vi "CSM - LogMem.vi"(5 "Init State(\"Macro: Initialize\")":string="Macro: Initialize", 7 "Name(\"\" to use uuid)":string="CSM Tiny") -> ()   [LabVIEW 2020]
doc: "Template for building CSM Module without User Interface.\n\n<b>Inputs:</b>\n- <b>Name(\"\" to use uuid)</b>: Module Name\n - If Input is \"\", an uuid will be used for module name. The module is marked as stand-alone mode and will not be included in module list.\n - Fi Input end with '#', the module will worked in worker mode. Modules with the same name will shared the same message queue. Any external message will be processed by one of the modules, depends on who is free.\n - Otherwise, the input string will be used as module name, which should be unique in system. CSM will go to \"Critical Error\" state if duplicated module name is used in system.\n\n<b>Outputs:</b>\n - N/A"
uses:
  <userlib>/_NEVSTOP/Communicable State Machine(CSM)/_Support/Priority Queue/Priority Queue.lvclass/Priority Queue.ctl
  Typedef/Def - Parsed CSMLog Line - Cluster.ctl
  ad4abf47-66ac-4882-9a91-90711142f294.vi
  aef905fb-f936-4b34-a29e-bd534a28b448.vi
  2c41bf92-7bf3-4770-9d59-94bc44f1e033.vi
  488b24ec-a7c0-4bee-a5e9-5f8eec7386e2.vi
  <userlib>/_NEVSTOP/Communicable State Machine(CSM)/_Support/Process/CSMP-Async Call.vi
  <userlib>/_NEVSTOP/Communicable State Machine(CSM)/_Support/GlobalEvent/GEvt-Generate Status Log.vi
  <userlib>/_NEVSTOP/Communicable State Machine(CSM)/_Support/Process/CSMP-Broadcast.vi
  <userlib>/_NEVSTOP/Communicable State Machine(CSM)/_Support/GlobalEvent/GEvt-Generate Interrupt Log.vi
  <userlib>/_NEVSTOP/Communicable State Machine(CSM)/_Support/GlobalEvent/GEvt-Generate Register Log.vi
  <userlib>/_NEVSTOP/Communicable State Machine(CSM)/_Support/Process/CSMP-Register Status.vi
  <userlib>/_NEVSTOP/Communicable State Machine(CSM)/_Support/GlobalEvent/GEvt-Generate Unregister Log.vi
  <userlib>/_NEVSTOP/Communicable State Machine(CSM)/_Support/Process/CSMP-Unregister Status.vi
  <userlib>/_NEVSTOP/Communicable State Machine(CSM)/_Support/Process/CSMP-Sync Call.vi
  <userlib>/_NEVSTOP/Communicable State Machine(CSM)/_Support/CSMQ/_CSMObj-Unlock.vi
  <userlib>/_NEVSTOP/Communicable State Machine(CSM)/_Support/Process/CSMP-PostPostMsg.vi
  <userlib>/_NEVSTOP/Communicable State Machine(CSM)/_Support/Process/CSMP-PostSendMsg.vi
  <userlib>/_NEVSTOP/Communicable State Machine(CSM)/_Support/CSMQ/_CSMObj-Lock State.vi
  <userlib>/_NEVSTOP/Communicable State Machine(CSM)/_Support/Common/Splite Reason String Part.vi
  <userlib>/_NEVSTOP/Communicable State Machine(CSM)/_Support/Common/Trim Single line Text.vi
  <userlib>/_NEVSTOP/Communicable State Machine(CSM)/_Support/CSMQ/_CSMOFGV Release.vi
  <userlib>/_NEVSTOP/Communicable State Machine(CSM)/_Support/Common/Remove Comments from Line.vi
  <userlib>/_NEVSTOP/Communicable State Machine(CSM)/_Support/Common/Splite Single-line Message.vi
  <userlib>/_NEVSTOP/Communicable State Machine(CSM)/_Support/Common/Parse Next Single-line State.vi
  <userlib>/_NEVSTOP/Communicable State Machine(CSM)/_Support/CSMQ/_CSMOFGV Dequeue.vi
  <userlib>/_NEVSTOP/Communicable State Machine(CSM)/_Support/CSMQ/_CSMObj-Log Error if in a Remote Session.vi
  <userlib>/_NEVSTOP/Communicable State Machine(CSM)/_Support/GlobalEvent/GEvt-Generate State Change Log.vi
  <userlib>/_NEVSTOP/Communicable State Machine(CSM)/_Support/GlobalEvent/GEvt-Generate Remaining States Log.vi
  <userlib>/_NEVSTOP/Communicable State Machine(CSM)/_Support/GlobalEvent/GEvt-Generate Module Destroyed Log.vi
  <userlib>/_NEVSTOP/Communicable State Machine(CSM)/_Support/GlobalEvent/GEvt-Generate Complete Log.vi
  <userlib>/_NEVSTOP/Communicable State Machine(CSM)/_Support/GlobalEvent/GEvt-Generate Module Created Log.vi
  <userlib>/_NEVSTOP/Communicable State Machine(CSM)/_Support/Common/Format Timestamp.vi
  <userlib>/_NEVSTOP/Communicable State Machine(CSM)/AdvanceAPI/CSM - Revert Arguments-Safe String.vi
  <userlib>/_NEVSTOP/Communicable State Machine(CSM)/AdvanceAPI/CSM - Make String Arguments Safe.vi
  <userlib>/_NEVSTOP/Communicable State Machine(CSM)/AdvanceAPI/CSM - Break Down Multiple States String.vi
  <userlib>/_NEVSTOP/Communicable State Machine(CSM)/AdvanceAPI/CSM - Compact Multiple States.vi
  <userlib>/_NEVSTOP/Communicable State Machine(CSM)/_Support/CSMQ/_CSMObj-Message Check.vi
  <userlib>/_NEVSTOP/Communicable State Machine(CSM)/_Support/CSMQ/_CSMObj-Enqueue Cross-Module Message.vi
  <userlib>/_NEVSTOP/Communicable State Machine(CSM)/_Support/CSMQ/_CSMOFGV Get.vi
  <userlib>/_NEVSTOP/Communicable State Machine(CSM)/_Support/FGV-BroadcastRegistry/Cache-Broadcast Registry Search Result.vi
  <userlib>/_NEVSTOP/Communicable State Machine(CSM)/AdvanceAPI/CSM - Register Status Change.vi
  <userlib>/_NEVSTOP/Communicable State Machine(CSM)/AdvanceAPI/CSM - Unregister Status Change.vi
  <userlib>/_NEVSTOP/Communicable State Machine(CSM)/_Support/Common/Hex Str to U8 Data.vi
  <userlib>/_NEVSTOP/Communicable State Machine(CSM)/_Support/Common/Concatenate State with Arguments.vi
  <userlib>/_NEVSTOP/Communicable State Machine(CSM)/_Support/Common/U8 Data to Hex Str.vi
  <userlib>/_NEVSTOP/Communicable State Machine(CSM)/_Support/Priority Queue/Dequeue Element.vi
  <userlib>/_NEVSTOP/Communicable State Machine(CSM)/AdvanceAPI/CSM - Keywords.vi
  <userlib>/_NEVSTOP/Communicable State Machine(CSM)/_Support/Priority Queue/Enqueue Element.vi
  <userlib>/_NEVSTOP/Communicable State Machine(CSM)/Utility/Trim Both Whitespace.vi
  <userlib>/_NEVSTOP/Communicable State Machine(CSM)/_Support/GlobalEvent/FGV-GlobalEventRef.vi
  <userlib>/_NEVSTOP/Communicable State Machine(CSM)/_Support/CSMQ/_CSMOFGV Obtain.vi
  <userlib>/_NEVSTOP/Communicable State Machine(CSM)/_Support/CSMQ/_CSMOFGV.vi
  <userlib>/_NEVSTOP/Communicable State Machine(CSM)/_Support/Error/CSM Not Allowed Message.vi
  <userlib>/_NEVSTOP/Communicable State Machine(CSM)/_Support/GlobalEvent/FGV-StatusChangeEventRef.vi
  <userlib>/_NEVSTOP/Communicable State Machine(CSM)/_Support/FGV-BroadcastRegistry/global-CSMQ FGV Change Flag.vi
  <userlib>/_NEVSTOP/Communicable State Machine(CSM)/_Support/FGV-BroadcastRegistry/global-Broadcast Cache Change Flag.vi
  <userlib>/_NEVSTOP/Communicable State Machine(CSM)/_Support/BroadcastRegistry/HelperVI/Broadcast Item Key.vi
  <userlib>/_NEVSTOP/Communicable State Machine(CSM)/_Support/FGV-BroadcastRegistry/FGV-BroadcastRegistry.vi
  <userlib>/_NEVSTOP/Communicable State Machine(CSM)/_Support/Message/Parse Register Message.vi
  <userlib>/_NEVSTOP/Communicable State Machine(CSM)/_Support/Message/Parse Unregister Message.vi
  <userlib>/_NEVSTOP/Communicable State Machine(CSM)/addons/API-String-Arugments-Support/_Support/Convert API String Arguments to Data(variant).vi
  <userlib>/_NEVSTOP/Communicable State Machine(CSM)/addons/MassData-Parameter/_support/FGV-MassData.vi
  <userlib>/_NEVSTOP/Communicable State Machine(CSM)/addons/API-String-Arugments-Support/_Support/Data To API String Arguments.vi
  <userlib>/_NEVSTOP/Communicable State Machine(CSM)/Communicable State Machine.lvlib
  <userlib>/_NEVSTOP/Communicable State Machine(CSM)/addons/Loop-Support/CSM Loop Support.lvlib
panel:
  out "size(s)":i32
  out "temp":string[](array[string])
  out "Snippets Count":i32
  out "State History":string
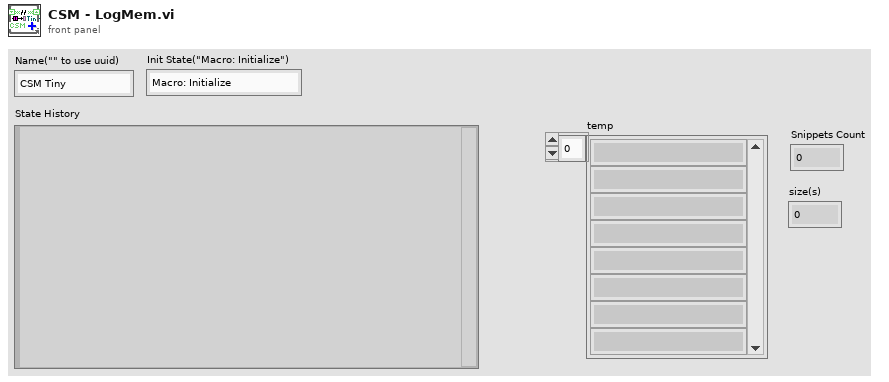
[diagram p1: front panel]
types:
  T1 = enum32{"Invalid", "Standard", "Closed", "Hidden", "Minimized", "Maximized"}
  T2 = enum32{"invalid app kind", "Development System", "Run Time System", "Student Edition", "Embedded LabVIEW", "Evaluation", "Custom"}
  T3 = typedef "Def - Parsed CSMLog Line - Cluster.ctl" = cluster{"Timestamp":timestamp, "Log Type":string, "CSM":string, "Log":string, "RawString":string}
  T4 = typedef "Communicable State Machine.lvlib/_CSM_Response Source Message.ctl" = cluster{"‘State":string, "’Arguments":string, "’Error":errorcluster}
  T5 = cluster{"Core":cluster{"Current VI Reference":refnum<vi>, "Close Panel on Exit?":bool}, "temp":string[], "Snippets Count":i32, "data":T3[]}
  T6 = cluster{"Current VI Reference":refnum<vi>, "Close Panel on Exit?":bool}
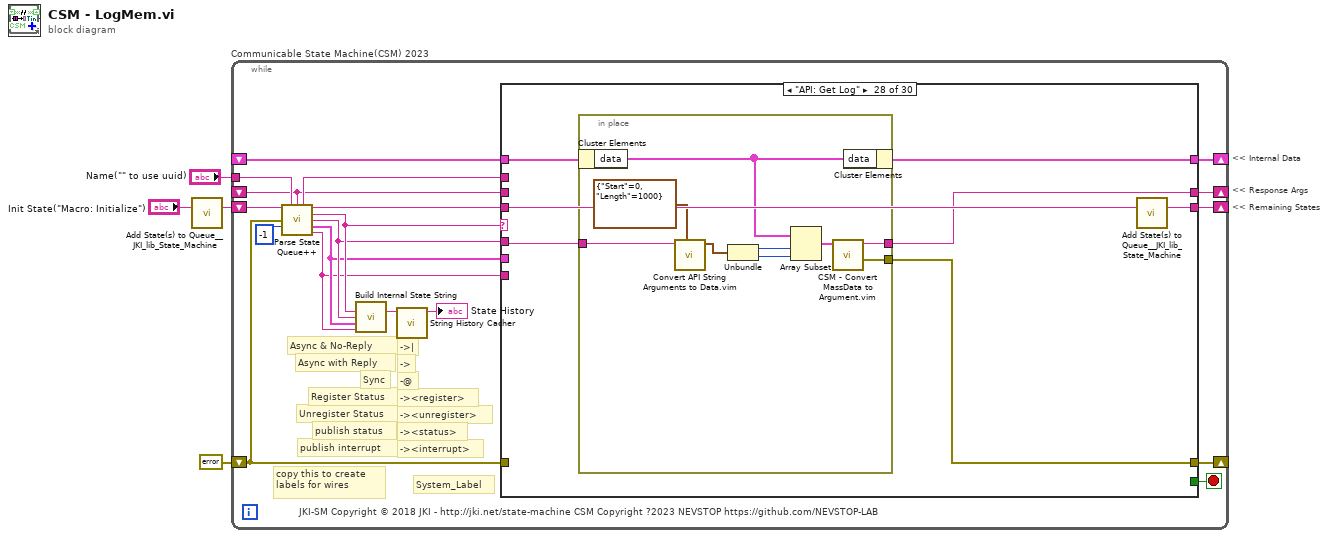
[diagram p0: block diagram]
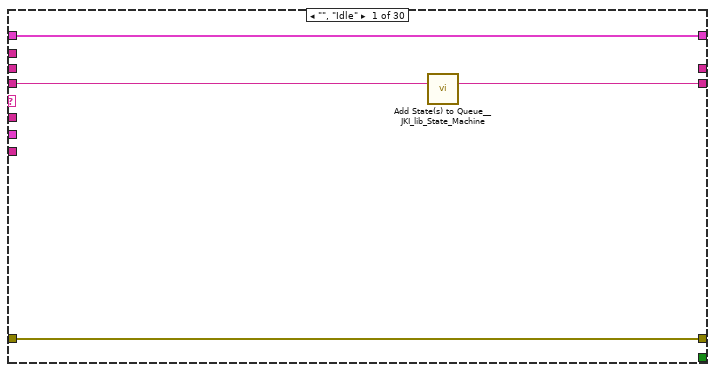
[diagram p2: hidden frame]
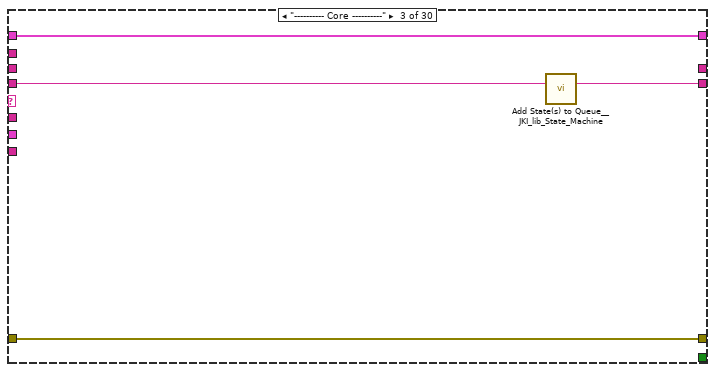
[diagram p4: hidden frame]
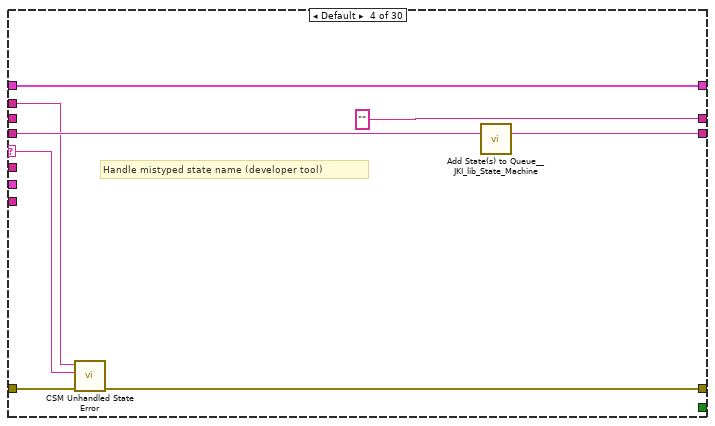
[diagram p5: hidden frame]
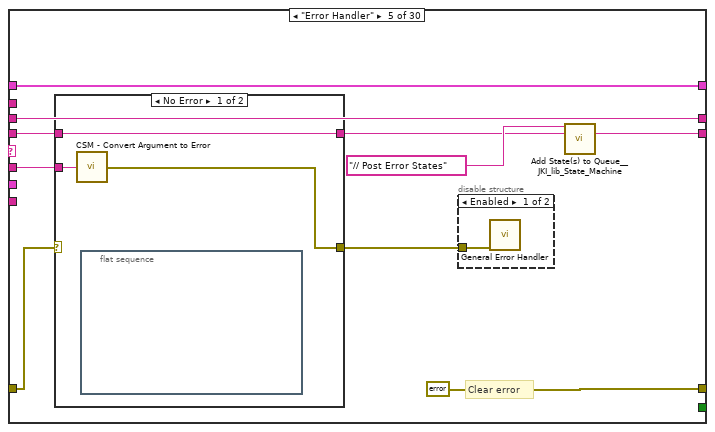
[diagram p6: hidden frame]
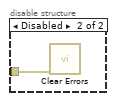
[diagram p7: hidden frame]
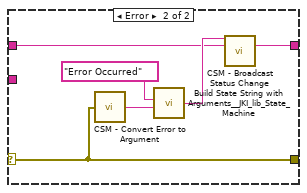
[diagram p8: hidden frame]
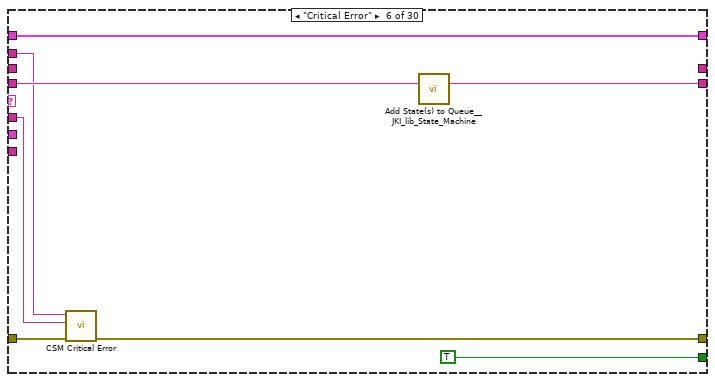
[diagram p9: hidden frame]
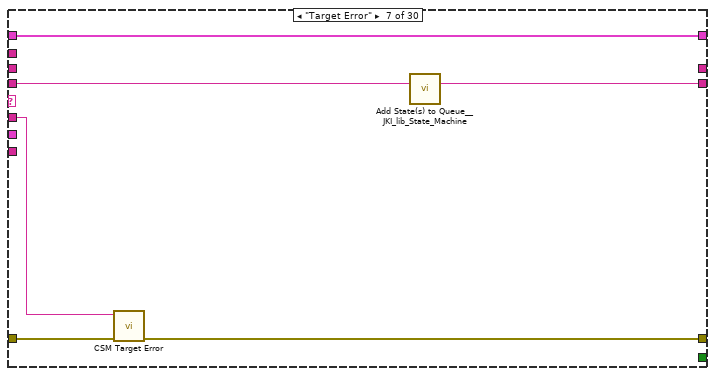
[diagram p10: hidden frame]
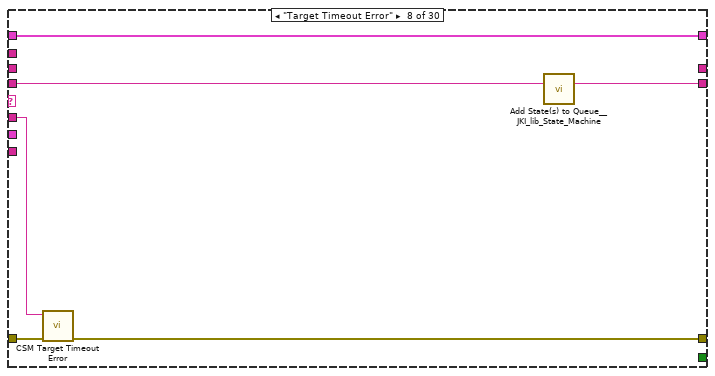
[diagram p11: hidden frame]
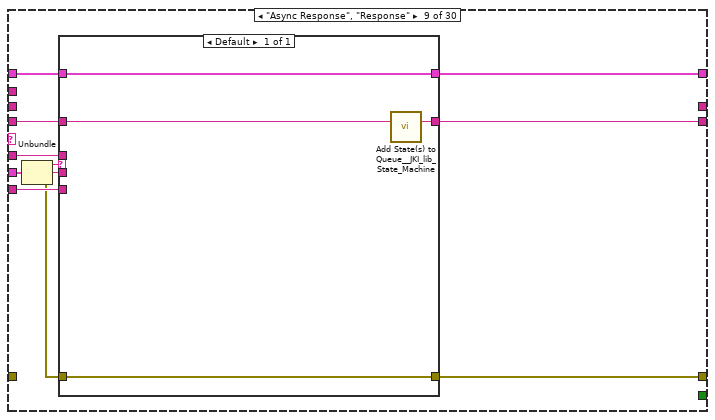
[diagram p12: hidden frame]
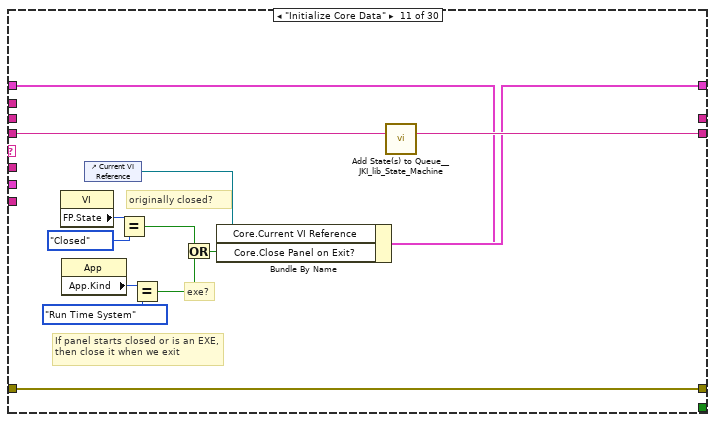
[diagram p14: hidden frame]
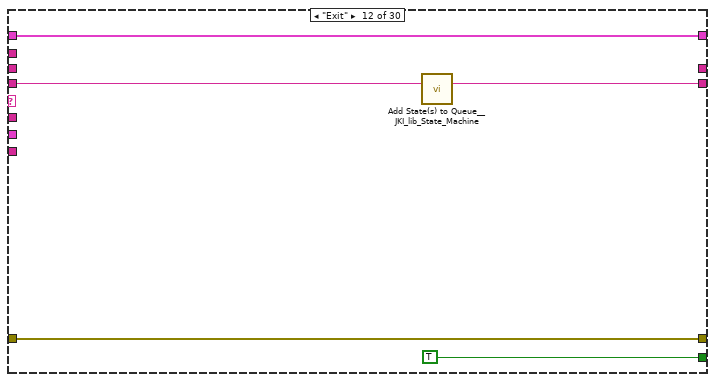
[diagram p15: hidden frame]
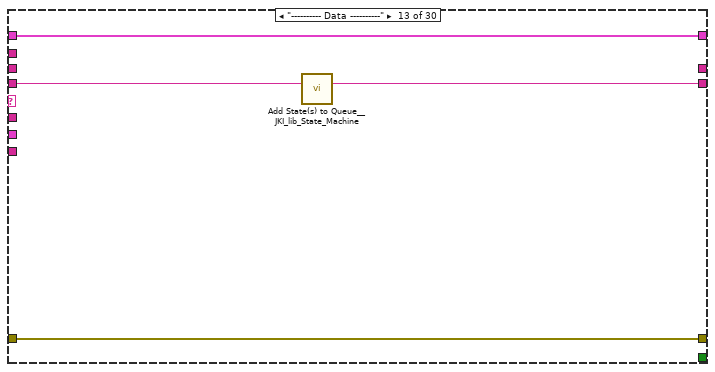
[diagram p16: hidden frame]
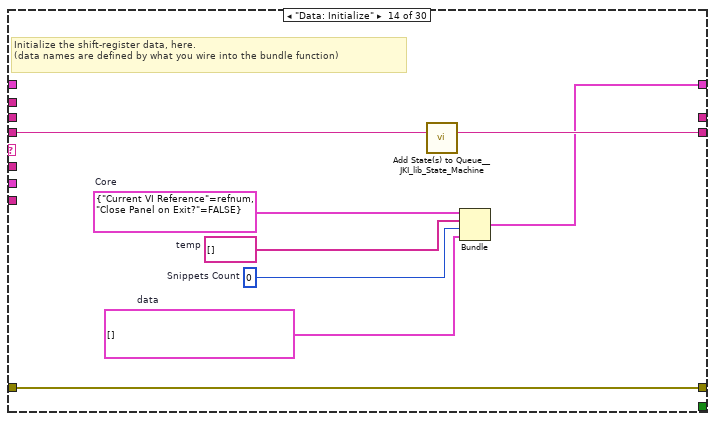
[diagram p17: hidden frame]
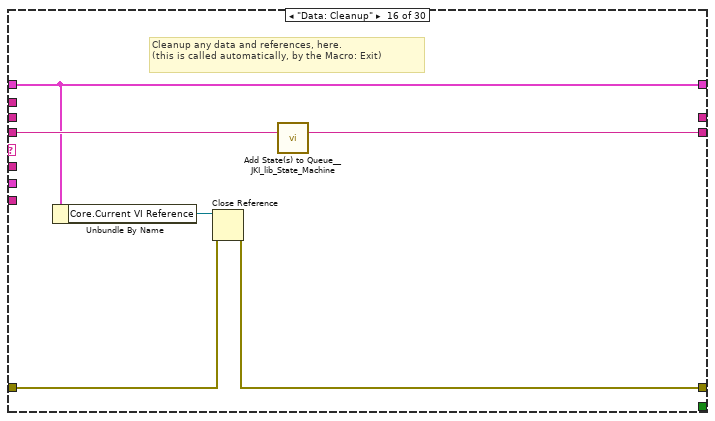
[diagram p19: hidden frame]
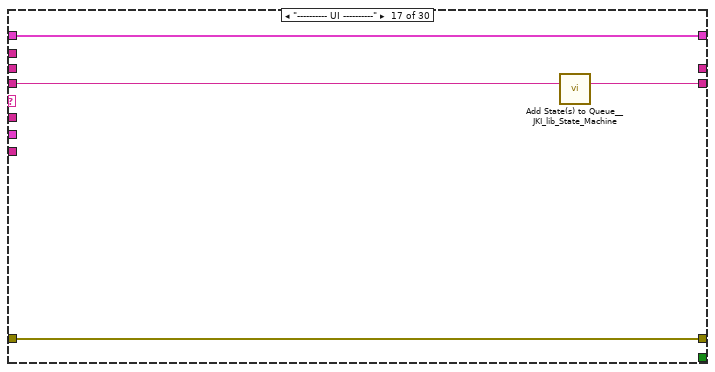
[diagram p20: hidden frame]
diagram:
  # "<< Internal Data"
  # "<< Response Args"
  # "<< Remaining States"
  n1 = call <vilib>:"Add State(s) to Queue__JKI_lib_State_Machine.vi"("State(s) in (\"\")"="Init State(\"Macro: Initialize\")") -> ("States Out"=w4:string)  [unwired: 14 in]
  n2 = while "Communicable State Machine(CSM) 2023" {
    shift-right: [w18] -> _
    shift-left: _ -> [w17]
    shift-right: [w21] -> _
    shift-left: errorcluster {"status"=FALSE, "code"=0, "source"=""} ("error out") -> [w16]
    shift-right: [w20] -> _
    shift-left: w4 -> [w22]
    tunnel: "Name(\"\" to use uuid)" -> [w14]
    shift-right: [w15] -> _
    shift-left: _ -> [w6]
    stop <- w19 stop-if-true
    # "-><interrupt>"
    # "-><status>"
    # "-><unregister>"
    # "-><register>"
    # "-@"
    # "->"
    # "->|"
    # "publish interrupt"
    # "publish status"
    # "Unregister Status"
    # "Register Status"
    # "Sync"
    # "Async with Reply"
    # "Async & No-Reply"
    # "copy this to create labels for wires"
    # "System_Label"
    # "JKI-SM Copyright © 2018 JKI - http://jki.net/state-machine CSM Copyright ?2023 NEVSTOP https://github.com/NEVSTOP-LAB"
    n3 = call <userlib>:"Parse State Queue++.vi"("State Queue"=w22, "Name(\"\" to use uuid)"=w14, "Response Arguments"=w6, "Error In (no error)"=w16, "Dequeue Timeout(0ms)"=-1 ("Timeout")) -> ("Name Used"=w7:string, "Remaining States"=w23:string, "Current State"=w11:string, "Arguments"=w10:string, ">> Response Source Message >>"=w9:T4, ">> Source CSM >>"=w8:string)  [unwired: 5 in]
    n4 = call <userlib>:"Build Internal State String.vi"("State"=w11, "Arguments (\"\")"=w10, ">> Response Source Message >>"=w9, "Source (\"\")"=w8) -> ("State with Arguments"=w12:string)  [unwired: 11 in]
    n5 = call <userlib>:"String History Cacher.vi"("String"=w12) -> ("String Cache"=→"State History":string)  [unwired: 10 in]
    n6 = case shown="\"API: Get Log\"" w11 {
      selector: w11 -> [_ _ _ w37 _ _ _ _ _ _ _ _ _ _ _ _ _ _ _ _ _ _ _ _ _ _ _ _ _ _]
      tunnel: w23 -> [w24 w29 w34 w41 w48 w69 w75 w81 w89 w100 w114 w119 w123 w131 w133 w140 w144 w148 w154 w169 w238 w243 w250 w252 w259 w262 w272 w283 w299 w300]
      tunnel: w10 -> [_ _ _ _ w47 w65 w74 w79 w88 _ _ _ _ _ _ _ _ _ w149 w163 _ _ _ _ _ w264 _ w280 _ _]
      tunnel: w17 -> [w25 w28 w31 w39 w51 w70 w76 w82 w91 w99 w107 w117 w120 _ w132 w135 w141 w146 w152 w165 w235 w240 w247 w251 w258 w266 w275 w286 w296 w302]
      tunnel: [w26 w30 w32 w35 errorcluster {"status"=FALSE, "code"=0, "source"=""} ("error out") w66 w72 w78 w94 w101 w111 w116 w121 w128 w134 w136 w142 w145 w150 w166 w236 w241 w248 w253 w260 _ w270 w281 w297 _] -> w21
      tunnel: w16 -> [w26 w30 w32 w42 w49 w71 w73 w80 _ w101 w111 w116 w121 w128 w134 w137 w142 w145 w151 w167 w236 w241 w248 w253 w260 _ _ _ w297 _]
      tunnel: [w27 w29 w33 w40 w44 w68 w77 w83 w90 w100 w113 w118 w122 w130 w133 w139 w143 w147 w153 w168 w237 w242 w249 w252 w257 w263 w273 w284 w298 w300] -> w20
      tunnel: [_ _ _ _ _ TRUE _ _ _ _ _ TRUE _ _ _ _ _ _ _ _ _ _ _ _ _ _ _ _ _ _] -> w19
      tunnel: [w25 w28 w31 w39 w51 w70 w76 w82 w92 w99 w112 w117 w120 w129 w132 w135 w141 w146 w152 w165 w235 w240 w247 w251 w256 w265 w274 w285 w296 w301] -> w18
      tunnel: w8 -> [_ _ _ _ _ _ _ _ w86 _ _ _ _ _ _ _ _ _ _ _ _ _ _ _ _ _ _ _ _ _]
      tunnel: w9 -> [_ _ _ _ _ _ _ _ w93 _ _ _ _ _ _ _ _ _ _ _ _ _ _ _ _ _ _ _ _ _]
      tunnel: [_ _ _ "" w43 _ _ _ _ _ _ _ _ _ _ _ _ _ _ _ _ _ _ _ _ _ w271 w282 _ _] -> w15
      tunnel: w7 -> [_ _ _ w36 _ w64 _ _ _ _ _ _ _ _ _ _ _ _ _ _ _ _ _ _ _ _ _ _ _ _]
      tunnel: w6 -> [_ _ _ _ w43 _ _ _ _ _ _ _ _ _ _ _ _ _ _ _ _ _ _ _ _ _ _ _ _ _]
      frame "", "Idle" {
        n7 = call <vilib>:"Add State(s) to Queue__JKI_lib_State_Machine.vi"("State(s) in (\"\")"=w24) -> ("States Out"=w27:string)  [unwired: 14 in]
      }
      frame "CSM Documentation" {
      }
      frame "---------- Core ----------" {
        n8 = call <vilib>:"Add State(s) to Queue__JKI_lib_State_Machine.vi"("State(s) in (\"\")"=w34) -> ("States Out"=w33:string)  [unwired: 14 in]
      }
      frame Default {
        # "Handle mistyped state name (developer tool)"
        n9 = call <userlib>:"CSM Unhandled State Error.vi"("error in (no error)"=w42, "State"=w37, "CSM"=w36) -> ("error out"=w35:errorcluster)  [unwired: 8 in]
        n10 = call <vilib>:"Add State(s) to Queue__JKI_lib_State_Machine.vi"("State(s) in (\"\")"=w41) -> ("States Out"=w40:string)  [unwired: 14 in]
      }
      frame "Error Handler" {
        # "Clear error"
        n11 = case shown="No Error" w49 {
          selector: w49 -> [_ w58]
          tunnel: [w57 w60] -> w45
          tunnel: w48 -> [w57 w59]
          tunnel: w47 -> [w56 _]
          tunnel: [w55 w58] -> w50
          frame No Error {
            n12 = call <userlib>:"CSM - Convert Argument to Error.vi"("Argument"=w56) -> ("error"=w55:errorcluster)  [unwired: 4 in]
            n13 = flat-sequence {
              frame #0 {
              }
            }
          }
          frame Error {
            n14 = call <userlib>:"CSM - Convert Error to Argument.vi"("error in (no error)"=w58) -> ("Arguments"=w62:string)  [unwired: 4 in]
            n15 = call <vilib>:"Build State String with Arguments__JKI_lib_State_Machine.vi"("Arguments (\"\")"=w62, "State"="Error Occurred" ("Status with Arguments")) -> ("State with Arguments"=w61:string)  [unwired: 4 in]
            n16 = call <userlib>:"CSM - Broadcast Status Change.vi"("Status with Arguments"=w61, "State Queue"=w59) -> ("Remaining States"=w60:string)  [unwired: 13 in]
          }
        }
        n17 = disable-structure shown="Enabled" {
          disable-tunnel: w50 -> [w53 w54]
          frame Enabled {
            n18 = call <vilib>:"General Error Handler.vi"("error in (no error)"=w53) -> ()  [unwired: 10 in, 5 out]
          }
          frame Disabled {
            n19 = call <vilib>:"Clear Errors.vi"("error in (no error)"=w54) -> ()  [unwired: 5 in, 2 out]
          }
        }
        n20 = call <vilib>:"Add State(s) to Queue__JKI_lib_State_Machine.vi"("State(s) in Front (\"\")"="// Post Error States", "State(s) in (\"\")"=w45) -> ("States Out"=w44:string)  [unwired: 13 in]
      }
      frame "Critical Error" {
        n21 = call <userlib>:"CSM Critical Error.vi"("error in (no error)"=w71, "input"=w65, "CSM Name"=w64) -> ("error out"=w66:errorcluster)  [unwired: 8 in]
        n22 = call <vilib>:"Add State(s) to Queue__JKI_lib_State_Machine.vi"("State(s) in (\"\")"=w69) -> ("States Out"=w68:string)  [unwired: 14 in]
      }
      frame "Target Error" {
        n23 = call <userlib>:"CSM Target Error.vi"("error in (no error)"=w73, "CSM Name"=w74) -> ("error out"=w72:errorcluster)  [unwired: 9 in]
        n24 = call <vilib>:"Add State(s) to Queue__JKI_lib_State_Machine.vi"("State(s) in (\"\")"=w75) -> ("States Out"=w77:string)  [unwired: 14 in]
      }
      frame "Target Timeout Error" {
        n25 = call <userlib>:"CSM Target Timeout Error.vi"("error in (no error)"=w80, "CSM Name"=w79) -> ("error out"=w78:errorcluster)  [unwired: 9 in]
        n26 = call <vilib>:"Add State(s) to Queue__JKI_lib_State_Machine.vi"("State(s) in (\"\")"=w81) -> ("States Out"=w83:string)  [unwired: 14 in]
      }
      frame "Async Response", "Response" {
        n27 = Unbundle(w93) -> ("‘State"=w87:string, "’Arguments"=w85:string, "’Error"=w84:errorcluster)
        n28 = case shown="Default" w87 {
          tunnel: [w98] -> w94
          tunnel: w84 -> [w98]
          tunnel: [w97] -> w92
          tunnel: w91 -> [w97]
          tunnel: [w95] -> w90
          tunnel: w89 -> [w96]
          tunnel: w88 -> [_]
          tunnel: w86 -> [_]
          tunnel: w85 -> [_]
          frame Default {
            n29 = call <vilib>:"Add State(s) to Queue__JKI_lib_State_Machine.vi"("State(s) in (\"\")"=w96) -> ("States Out"=w95:string)  [unwired: 14 in]
          }
        }
      }
      frame "Async Message Posted" {
      }
      frame "Initialize Core Data" {
        # "originally closed?"
        # "exe?"
        # "If panel starts closed or is an EXE, then close it when we exit"
        n30 = property class="VI"() -> ("FP.State"=w104:T1)  [unwired: 2 in, 2 out]
        n31 = property class="App"() -> ("App.Kind"=w110:T2)  [unwired: 2 in, 2 out]
        n32 = control-ref of="Current VI Reference"() -> (w105:refnum<vi>)
        n33 = Equal?(x=w104, y=T1."Closed" ("Front Panel Window:State")) -> (x = y?=w102:bool)
        n34 = Equal?(x=w110, y=T2."Run Time System" ("Application:Kind")) -> (x = y?=w108:bool)
        n35 = Or(x=w102, y=w108) -> (x .or. y?=w106:bool)
        n36 = Bundle By Name(cluster=w107, "Core.Current VI Reference"=w105, "Core.Close Panel on Exit?"=w106) -> (w112:T5)
        n37 = call <vilib>:"Add State(s) to Queue__JKI_lib_State_Machine.vi"("State(s) in (\"\")"=w114) -> ("States Out"=w113:string)  [unwired: 14 in]
      }
      frame "Exit" {
        n38 = call <vilib>:"Add State(s) to Queue__JKI_lib_State_Machine.vi"("State(s) in (\"\")"=w119) -> ("States Out"=w118:string)  [unwired: 14 in]
      }
      frame "---------- Data ----------" {
        n39 = call <vilib>:"Add State(s) to Queue__JKI_lib_State_Machine.vi"("State(s) in (\"\")"=w123) -> ("States Out"=w122:string)  [unwired: 14 in]
      }
      frame "Data: Initialize" {
        w124 = T3[] []  # data
        w125 = 0  # Snippets Count
        w126 = string[] []  # temp
        w127 = T6 {"Current VI Reference"=refnum, "Close Panel on Exit?"=FALSE}  # Core
        # "Initialize the shift-register data, here.\n(data names are defined by what you wire into the bundle function)"
        n40 = call <vilib>:"Add State(s) to Queue__JKI_lib_State_Machine.vi"("State(s) in (\"\")"=w131) -> ("States Out"=w130:string)  [unwired: 14 in]
        n41 = Bundle("Core"=w127, "temp"=w126, "Snippets Count"=w125, "data"=w124) -> (w129:T5)  [unwired: 1 in]
      }
      frame "Data: Update Indicators" {
      }
      frame "Data: Cleanup" {
        # "Cleanup any data and references, here.\n(this is called automatically, by the Macro: Exit)"
        n42 = Unbundle By Name(w135) -> ("Core.Current VI Reference"=w138:refnum<vi>)
        n43 = Close Reference(reference=w138, error in (no error)=w137) -> (error out=w136:errorcluster)
        n44 = call <vilib>:"Add State(s) to Queue__JKI_lib_State_Machine.vi"("State(s) in (\"\")"=w140) -> ("States Out"=w139:string)  [unwired: 14 in]
      }
      frame "---------- UI ----------" {
        n45 = call <vilib>:"Add State(s) to Queue__JKI_lib_State_Machine.vi"("State(s) in (\"\")"=w144) -> ("States Out"=w143:string)  [unwired: 14 in]
      }
      frame "UI: Initialize" {
        n46 = call <vilib>:"Add State(s) to Queue__JKI_lib_State_Machine.vi"("State(s) in (\"\")"=w148) -> ("States Out"=w147:string)  [unwired: 14 in]
      }
      frame "UI: Cursor Set" {
        # "Argument"
        n47 = disable-structure shown="TARGET_TYPE!=Windows" {
          disable-tunnel: w151 -> [w157 w162]
          disable-tunnel: [w156 w162] -> w150
          disable-tunnel: w149 -> [w155 _]
          frame condition #0 (active) {
            n48 = case shown="\"Idle\", Default" w155 {
              tunnel: w157 -> [w159 w161]
              tunnel: [w158 w160] -> w156
              frame "Idle", Default {
                n49 = call <vilib>:"Unset Busy.vi"("error in (no error)"=w159) -> ("error out"=w158:errorcluster)  [unwired: 10 in]
              }
              frame "Busy" {
                n50 = call <vilib>:"Set Busy.vi"("error in (no error)"=w161) -> ("error out"=w160:errorcluster)  [unwired: 9 in, 1 out]
              }
            }
          }
          frame condition #1 {
          }
        }
        n51 = call <vilib>:"Add State(s) to Queue__JKI_lib_State_Machine.vi"("State(s) in (\"\")"=w154) -> ("States Out"=w153:string)  [unwired: 14 in]
      }
      frame "UI: Front Panel State" {
        # "Argument"
        n52 = Unbundle By Name(w165) -> ("Core.Current VI Reference"=w164:refnum<vi>)
        n53 = call <vilib>:"Add State(s) to Queue__JKI_lib_State_Machine.vi"("State(s) in (\"\")"=w169) -> ("States Out"=w168:string)  [unwired: 14 in]
        n54 = case shown="\"Close\", \"Closed\"" w163 {
          tunnel: w167 -> [w175 w190 w201 w214 w227]
          tunnel: [w177 w191 w203 w216 w229] -> w166
          tunnel: w164 -> [w176 w188 w202 w215 w228]
          frame "Open", "Standard", Default {
            w170 = T1."Standard" ("State")
            n55 = property class="VI"(reference=w176, error in=w175) -> (reference out=w173:refnum<vi>, error out=w174:errorcluster, "FP.State"=w172:T1)
            n56 = Not Equal?(x=w172, y=w170) -> (x != y?=w171:bool)
            n57 = case shown="True" w171 {
              tunnel: [w181 w183] -> w177
              tunnel: w174 -> [w180 w183]
              tunnel: w173 -> [w179 _]
              tunnel: w170 -> [w178 _]
              frame True {
                n58 = invoke class="VI" method="FP.Open"(reference=w179, error in=w180, "Activate"=TRUE, "State"=w178) -> (error out=w181:errorcluster)  [unwired: 1 in, 4 out]
              }
              frame False {
              }
            }
          }
          frame "Close", "Closed" {
            n59 = property class="VI"(reference=w188, error in=w190) -> (reference out=w187:refnum<vi>, error out=w189:errorcluster, "FP.State"=w185:T1)
            n60 = Not Equal?(x=w185, y=T1."Closed" ("Front Panel Window:State")) -> (x != y?=w184:bool)
            n61 = case shown="False" w184 {
              tunnel: [w192 w195] -> w191
              tunnel: w189 -> [w192 w194]
              tunnel: w187 -> [_ w193]
              frame False {
              }
              frame True {
                n62 = invoke class="VI" method="FP.Close"(reference=w193, error in=w194) -> (error out=w195:errorcluster)  [unwired: 1 in, 2 out]
              }
            }
          }
          frame "Hidden", "Hide" {
            w196 = T1."Hidden" ("State")
            n63 = property class="VI"(reference=w202, error in=w201) -> (reference out=w199:refnum<vi>, error out=w200:errorcluster, "FP.State"=w198:T1)
            n64 = Not Equal?(x=w198, y=w196) -> (x != y?=w197:bool)
            n65 = case shown="True" w197 {
              tunnel: [w207 w208] -> w203
              tunnel: w200 -> [w206 w208]
              tunnel: w199 -> [w205 _]
              tunnel: w196 -> [w204 _]
              frame True {
                n66 = invoke class="VI" method="FP.Open"(reference=w205, error in=w206, "State"=w204) -> (error out=w207:errorcluster)  [unwired: 2 in, 4 out]
              }
              frame False {
              }
            }
          }
          frame "Minimize", "Minimized" {
            w209 = T1."Minimized" ("State")
            n67 = property class="VI"(reference=w215, error in=w214) -> (reference out=w212:refnum<vi>, error out=w213:errorcluster, "FP.State"=w211:T1)
            n68 = Not Equal?(x=w211, y=w209) -> (x != y?=w210:bool)
            n69 = case shown="True" w210 {
              tunnel: [w220 w221] -> w216
              tunnel: w213 -> [w219 w221]
              tunnel: w212 -> [w218 _]
              tunnel: w209 -> [w217 _]
              frame True {
                n70 = invoke class="VI" method="FP.Open"(reference=w218, error in=w219, "State"=w217) -> (error out=w220:errorcluster)  [unwired: 2 in, 4 out]
              }
              frame False {
              }
            }
          }
          frame "Maximize", "Maximized" {
            w222 = T1."Maximized" ("State")
            n71 = property class="VI"(reference=w228, error in=w227) -> (reference out=w225:refnum<vi>, error out=w226:errorcluster, "FP.State"=w224:T1)
            n72 = Not Equal?(x=w224, y=w222) -> (x != y?=w223:bool)
            n73 = case shown="True" w223 {
              tunnel: [w233 w234] -> w229
              tunnel: w226 -> [w232 w234]
              tunnel: w225 -> [w231 _]
              tunnel: w222 -> [w230 _]
              frame True {
                n74 = invoke class="VI" method="FP.Open"(reference=w231, error in=w232, "State"=w230) -> (error out=w233:errorcluster)  [unwired: 2 in, 4 out]
              }
              frame False {
              }
            }
          }
        }
      }
      frame "---------- Macro ----------" {
        n75 = call <vilib>:"Add State(s) to Queue__JKI_lib_State_Machine.vi"("State(s) in (\"\")"=w238) -> ("States Out"=w237:string)  [unwired: 14 in]
      }
      frame "Macro: Initialize" {
        n76 = call <vilib>:"Add State(s) to Queue__JKI_lib_State_Machine.vi"("State(s) in Front (\"\")"="Data: Initialize\nInitialize Core Data\nData: Update Indicators", "State(s) in (\"\")"=w243) -> ("States Out"=w242:string)  [unwired: 13 in]
      }
      frame "Macro: Exit" {
        n77 = call <vilib>:"Add State(s) to Queue__JKI_lib_State_Machine.vi"("State(s) in Front (\"\")"="//Exit Sub-Modules ", "State(s) at Back (\"\")"="Data: Cleanup\nExit") -> ("States Out"=w245:string)  [unwired: 13 in]
        n78 = call <userlib>:"CSMLS - Add Exit State(s) with Loop Check.vi"("States Out in"=w245, "Remaining States"=w250) -> ("States Out out"=w249:string)  [unwired: 13 in]
      }
      frame "---------- API ----------" {
      }
      frame "API: Clear" {
        w254 = T3[] []  # data
        n79 = Bundle By Name(cluster=w258, "Snippets Count"=0, "data"=w254) -> (w256:T5)
        n80 = call <vilib>:"Add State(s) to Queue__JKI_lib_State_Machine.vi"("State(s) in (\"\")"=w259) -> ("States Out"=w257:string)  [unwired: 14 in]
      }
      frame "Handler: Record Snippets" {
        n81 = in-place {
          in-place-border: w264 -> [w267]
          n82 = in-place-cluster #1(w266) -> ("temp"=w269:string[])
          n83 = Build Array (concatenate)(w269, w267) -> (w268:string[])
          n84 = in-place-cluster #1("temp"=w268) -> (w265:T5)
        }
        n85 = call <vilib>:"Add State(s) to Queue__JKI_lib_State_Machine.vi"("State(s) in Front (\"\")"="Action: Process Parsed Snippet" ("State(s) in Front (\"\")"), "State(s) in (\"\")"=w262) -> ("States Out"=w263:string)  [unwired: 13 in]
      }
      frame "API: Log Length" {
        n86 = in-place {
          in-place-border: [w277] -> w271
          in-place-border: [w276] -> w270
          n87 = in-place-cluster #2(w275) -> ("data"=w279:T3[])
          n88 = Array Size(array=w279) -> (size(s)=w278:i32)
          n89 = call "Convert Data To API String Arguments.vim"("data"=w278) -> ("error out"=w276:errorcluster, "String"=w277:string)  [unwired: 7 in]
          n90 = in-place-cluster #2("data"=w279) -> (w274:T5)
        }
        n91 = call <vilib>:"Add State(s) to Queue__JKI_lib_State_Machine.vi"("State(s) in (\"\")"=w272) -> ("States Out"=w273:string)  [unwired: 14 in]
      }
      frame "API: Get Log" {
        n92 = in-place {
          in-place-border: [w295] -> w282
          in-place-border: [w294] -> w281
          in-place-border: w280 -> [w290]
          n93 = in-place-cluster #3(w286) -> ("data"=w293:T3[])
          n94 = call "Convert API String Arguments to Data.vim"("Type"=cluster{"Start":i32, "Length":i32} {"Start"=0, "Length"=1000}, "String"=w290) -> ("Data"=w289:cluster{"Start":i32, "Length":i32})  [unwired: 6 in, 1 out]
          n95 = Unbundle(w289) -> ("Start"=w288:i32, "Length"=w287:i32)
          n96 = Array Subset(array=w293, index=w288, length=w287) -> (w292:T3[])
          n97 = call "CSM - Convert MassData to Argument.vim"("DBL"=w292) -> ("error out"=w294:errorcluster, "MassData Argument"=w295:string)  [unwired: 7 in]
          n98 = in-place-cluster #3("data"=w293) -> (w285:T5)
        }
        n99 = call <vilib>:"Add State(s) to Queue__JKI_lib_State_Machine.vi"("State(s) in (\"\")"=w283) -> ("States Out"=w284:string)  [unwired: 14 in]
      }
      frame "---------- Action ----------" {
        n100 = call <vilib>:"Add State(s) to Queue__JKI_lib_State_Machine.vi"("State(s) in (\"\")"=w299) -> ("States Out"=w298:string)  [unwired: 14 in]
      }
      frame "Action: Process Parsed Snippet" {
        n101 = in-place {
          n102 = in-place-cluster #4(w302) -> ("temp"=w308:string[], "Snippets Count"=w306:i32, "data"=w305:T3[])
          n103 = for {
            tunnel: [w318] -> w309 mode=indexing if=w310
            tunnel: w308 -> [w318] mode=indexing
            shift-right: [w315] -> w307
            shift-left: w306 -> [w314]
            shift-right: [w313] -> w304
            shift-left: w305 -> [w312]
            n104 = call "CSM - Convert Argument to MassData.vim"("Type"=cluster{"index":i32, "Data":T3[]} {"index"=0, "Data"=[]} ("output cluster"), "MassData Argument"=w318) -> ("Data"=w319:cluster{"index":i32, "Data":T3[]})  [unwired: 6 in, 1 out]
            n105 = Unbundle By Name(w319) -> ("index"=w317:i32, "Data"=w311:T3[])
            n106 = Equal?(x=w314, y=w317) -> (x = y?=w316:bool)
            n107 = case shown="True" w316 {
              tunnel: [w323 w327] -> w315
              tunnel: w314 -> [w323 w328]
              tunnel: [w322 w325] -> w313
              tunnel: w312 -> [w322 w326]
              tunnel: w311 -> [_ w324]
              tunnel: [TRUE _] -> w310
              frame False {
              }
              frame True {
                n108 = Increment(x=w328) -> (x+1=w327:i32)
                n109 = Build Array (concatenate)(w326, w324) -> (w325:T3[])
              }
            }
          }
          "Snippets Count" <- w307
          "temp" <- w309
          n110 = Array Size(array=w304) -> (size(s)=→"size(s)":i32)
          n111 = in-place-cluster #4("temp"=w309, "Snippets Count"=w307, "data"=w304) -> (w301:T5)
        }
      }
    }
  }
